vi "Bounding Box to Rectangle ROI (LV 2013 SP1) (SubVI).vi"(11 "Bounding Box":cluster{"x":sgl, "y":sgl}[](array[cluster])) -> (3 "ROI Descriptor":T1 {"Contours"."Type" items=["No Selection", "Point", "Line", "Rectangle", "Oval", "Polygon", "Freehand Region", "Annulus", "Unused2", "Unused3", "Broken Line", "Freehand Line", "Rotated Rectangle"]})   [LabVIEW 2016]
doc: "Takes Arrays of Matches and filters the Bounding Box for each match. Then prepares coordinates to match rectangle region to allow creating ROIs"
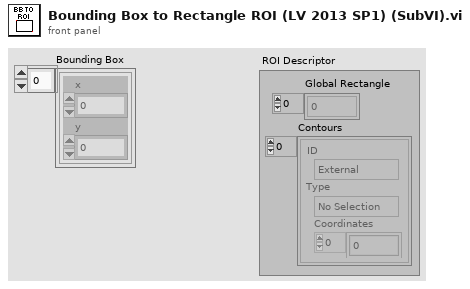
[diagram p1: front panel]
types:
  T1 = typedef "ROI Descriptor" = cluster{"Global Rectangle":i32[], "Contours":cluster{"ID":enum32{"External", "Internal"}, "Type":u32, "Coordinates":i32[]}[]}
  T2 = typedef "IMAQ Rectangle" = cluster{"Left":i32, "Top":i32, "Right":i32, "Bottom":i32, "Rotation":dbl}
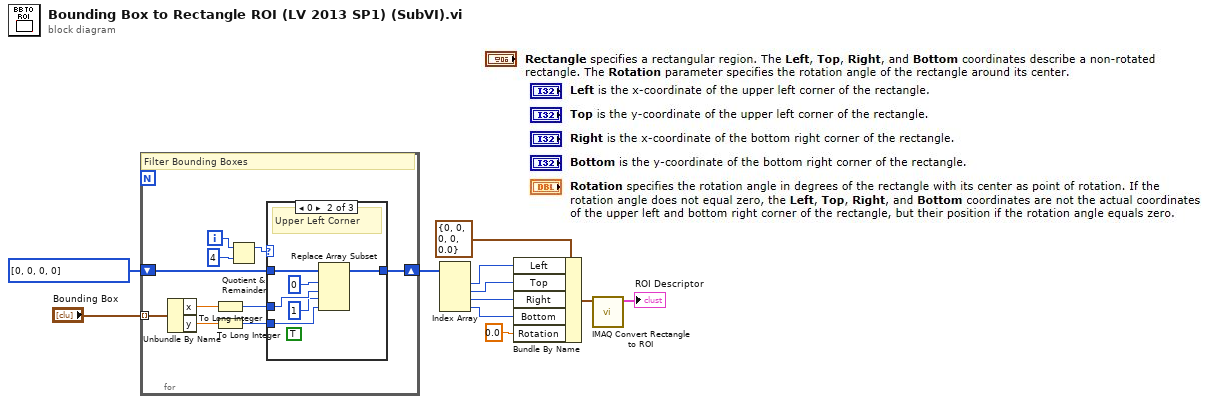
[diagram p0: block diagram]
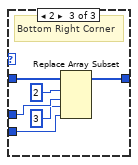
[diagram p3: hidden frame]
diagram:
  n1 = for {
    tunnel: "Bounding Box" -> [w14] mode=indexing
    shift-right: [w12] -> w4
    shift-left: i32[] [0, 0, 0, 0] -> [w13]
    i -> [w20]
    # "Filter Bounding Boxes"
    n2 = Unbundle By Name(w14) -> ("x"=w18:sgl, "y"=w19:sgl)
    n3 = To Long Integer(number=w18) -> (32bit integer=w17:i32)
    n4 = To Long Integer(number=w19) -> (32bit integer=w16:i32)
    n5 = Quotient & Remainder(x=w20, y=4) -> (x-y*floor(x/y)=w15:i32)  [unwired: 1 out]
    n6 = case shown="0" w15 {
      tunnel: w16 -> [_ w24 w30]
      tunnel: w17 -> [_ w26 w32]
      tunnel: w13 -> [w22 w28 w34]
      tunnel: [w22 w23 w29] -> w12
      frame -1, Default {
      }
      frame 0 {
        (unwired) TRUE
        # "Upper Left Corner"
        n7 = Replace Array Subset(array=w28, new element #1=w26, index #1=0, new element #2=w24, index #2=1) -> (w23:i32[])
      }
      frame 2 {
        # "Bottom Right Corner"
        n8 = Replace Array Subset(array=w34, new element #1=w32, index #1=2, new element #2=w30, index #2=3) -> (w29:i32[])
      }
    }
  }
  n9 = Index Array(array=w4) -> (element #1=w8:i32, element #2=w7:i32, element #3=w6:i32, element #4=w5:i32)  [unwired: 4 in]
  n10 = Bundle By Name(cluster=T2 {"Left"=0, "Top"=0, "Right"=0, "Bottom"=0, "Rotation"=0.0} ("Rectangle"), "Left"=w8, "Top"=w7, "Right"=w6, "Bottom"=w5, "Rotation"=0.0) -> (w2:T2)
  n11 = call "IMAQ Convert Rectangle to ROI"("Rectangle"=w2) -> ("ROI Descriptor"=→"ROI Descriptor":T1)  [unwired: 8 in, 1 out]
